vi "Control Inputs (SubVI).vi"(6 "Enable Kinect Extention":bool, 7 "Keyboard ID":refnum<k1>, 8 "error in (no error)":errorcluster, 9 "Switch control":bool, 10 "Manual":bool=TRUE, 11 "Controller ID":refnum<k1>) -> (0 "error out":errorcluster, 1 "Land/Take off":bool, 2 "Hover Out":bool, 3 "Control cluster":T1)   [LabVIEW 2014]
uses:
  Global.vi
panel:
  out "x-y":u32
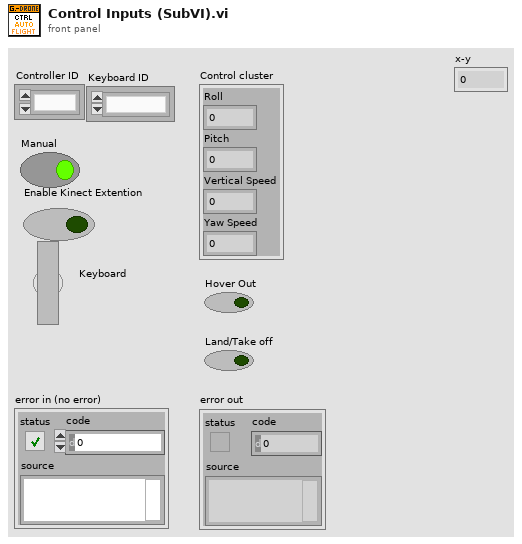
[diagram p1: front panel]
types:
  T1 = cluster{"Roll":dbl, "Pitch":dbl, "Vertical Speed":dbl, "Yaw Speed":dbl}
  T2 = cluster{"Hover":bool, "Land/Take off":bool, "button 3":bool, "button 4":bool}
  T3 = typedef "Control cluster.ctl" = cluster{"Roll":sgl, "Pitch":sgl, "Vertical Speed":sgl, "Yaw Speed":sgl}
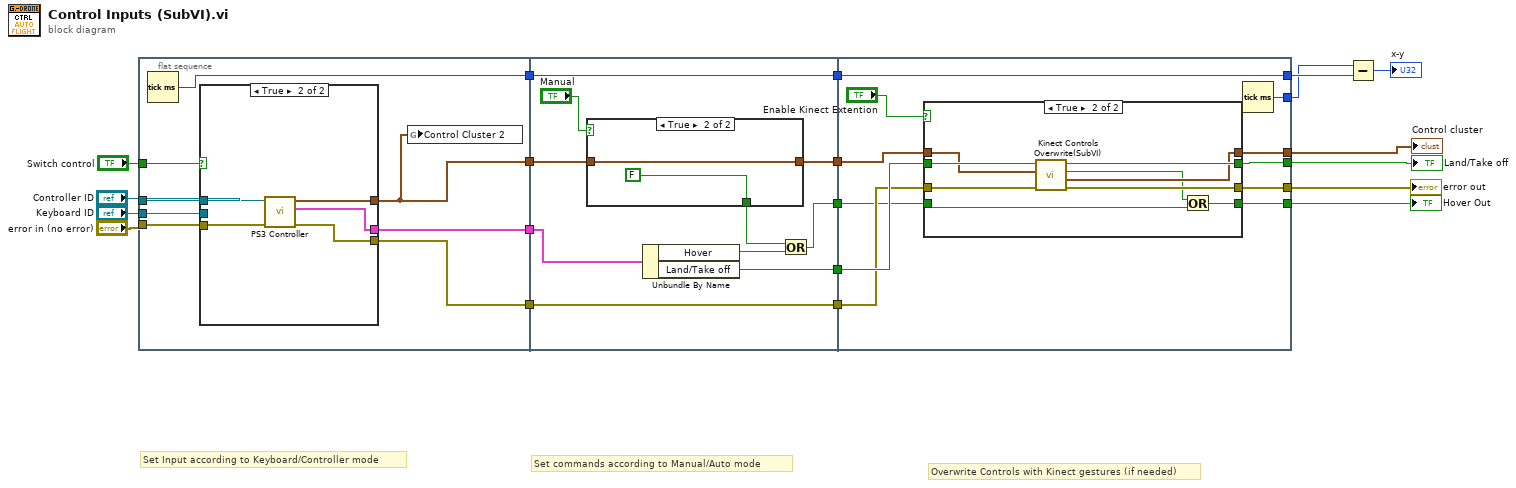
[diagram p0: block diagram]
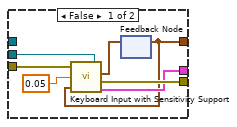
[diagram p2: hidden frame]
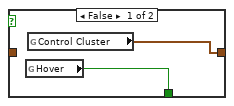
[diagram p3: hidden frame]
diagram:
  # "Overwrite Controls with Kinect gestures (if needed)"
  # "Set Input according to Keyboard/Controller mode"
  # "Set commands according to Manual/Auto mode"
  n1 = flat-sequence {
    tunnel: [w22] -> w14
    tunnel: [w26] -> w13
    tunnel: [w27] -> w12
    tunnel: "error in (no error)" -> [w28]
    tunnel: "Keyboard ID" -> [w25]
    tunnel: "Controller ID" -> [w24]
    tunnel: "Switch control" -> [w23]
    tunnel: [w21] -> w3
    tunnel: [w49] -> w20
    tunnel: [w47] -> w19
    tunnel: [w43] -> w18
    tunnel: [w42] -> w16
    tunnel: w14 -> [w50]
    tunnel: w13 -> [w46]
    tunnel: w12 -> [w43]
    tunnel: [w41] -> w4
    tunnel: w3 -> [w41]
    tunnel: w20 -> [w65]
    tunnel: w19 -> [w58]
    tunnel: w18 -> [w63]
    tunnel: [w62] -> w17
    tunnel: [w57] -> w6
    tunnel: w16 -> [w61]
    tunnel: [w60] -> w15
    tunnel: [w59] -> w7
    tunnel: [w56] -> w5
    tunnel: w4 -> [w56]
    tunnel: [w55] -> w2
    frame #0 {
      n2 = Tick Count (ms)() -> (millisecond timer value=w21:u32)
      n3 = case shown="True" w23 {
        tunnel: w28 -> [w35 w40]
        tunnel: [w34 w39] -> w27
        tunnel: [w30 w38] -> w22
        tunnel: [w33 w37] -> w26
        tunnel: w25 -> [w32 _]
        tunnel: w24 -> [_ w36]
        frame False {
          n4 = feedback #1() -> (w30:T1)  [unwired: 1 in]
          n5 = call "Keyboard Input with Sensitivity Support.vi"("error in (no error)"=w35, "Speed step"=0.05, "Previous Control Cluster"=w30, "device ID"=w32) -> ("Control Cluster"=w31:T1, "error out"=w34:errorcluster, "Buttons control"=w33:T2)
          n6 = feedback-in #1(w31) -> ()
        }
        frame True {
          n7 = call "PS3 Controller.vi"("error in (no error)"=w40, "device ID"=w36) -> ("error out"=w39:errorcluster, "Buttons control"=w37:T2, "Control cluster"=w38:T1)  [unwired: 7 in]
        }
      }
      n8 = global write "Global.vi" "Control Cluster 2"(w22) -> ()
    }
    frame #1 {
      n9 = case shown="True" "Manual" {
        tunnel: w50 -> [_ w53]
        tunnel: [w52 w53] -> w47
        tunnel: [w51 FALSE] -> w44
        frame False {
          n10 = global read "Global.vi" "Hover"() -> (w51:bool)
          n11 = global read "Global.vi" "Control Cluster"() -> (w52:T3)
        }
        frame True {
        }
      }
      n12 = Unbundle By Name(w46) -> ("Hover"=w45:bool, "Land/Take off"=w49:bool)
      n13 = Or(x=w44, y=w45) -> (x .or. y?=w42:bool)
    }
    frame #2 {
      n14 = case shown="True" "Enable Kinect Extention" {
        tunnel: w65 -> [w69 w78]
        tunnel: [w69 w77] -> w59
        tunnel: [w68 w76] -> w62
        tunnel: w63 -> [w68 w75]
        tunnel: w61 -> [w67 w70]
        tunnel: [w67 w72] -> w60
        tunnel: w58 -> [w66 w74]
        tunnel: [w66 w73] -> w57
        frame False {
        }
        frame True {
          n15 = call "Kinect Controls Overwrite(SubVI).vi"("error in (no error)"=w75, "Control cluster In"=w74, "Land/Take off In"=w78) -> ("error out"=w76:errorcluster, "Control cluster Out"=w73:T1, "Hover Out"=w71:bool, "Land/take off Out"=w77:bool)  [unwired: 5 in]
          n16 = Or(x=w71, y=w70) -> (x .or. y?=w72:bool)
        }
      }
      n17 = Tick Count (ms)() -> (millisecond timer value=w55:u32)
    }
  }
  n18 = Subtract(x=w2, y=w5) -> (x-y=→"x-y":u32)
  "error out" <- w17
  "Control cluster" <- w6
  "Land/Take off" <- w7
  "Hover Out" <- w15
